vi "TDS RF Signal Output Frequency.vi"(8 "error in (no error)":errorcluster, 9 "Frequency":dbl, 10 "Signal InstConfig":string, 11 "Address":string) -> (0 "error out":errorcluster)   [LabVIEW 2025, in "Interface Functions.lvlib"]
uses:
  Interface Functions.lvlib
panel:
  out "read buffer":string
  # "RF Signal Output Frequency"
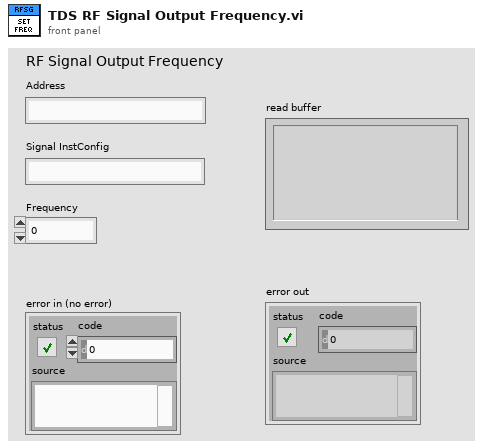
[diagram p1: front panel]
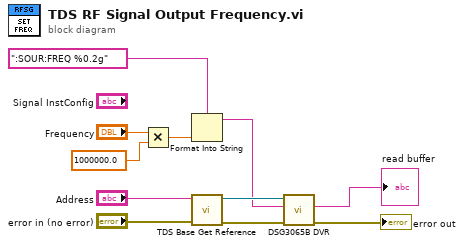
[diagram p0: block diagram]
diagram:
  n1 = Multiply(x="Frequency", y=1000000.0) -> (x*y=w1:dbl)
  n2 = Format Into String(format string=":SOUR:FREQ %0.2g", w1) -> (resulting string=w5:string)  [unwired: 2 in, 1 out]
  n3 = call "TDS Base Get Reference.vi"("error in (no error)"="error in (no error)", "Address"="Address") -> ("error out"=w8:errorcluster, "Reference"=w6:refnum<visa-resource-name>)  [unwired: 8 in]
  n4 = call "DSG3065B DVR.vi"("error in (no error)"=w8, "write buffer"=w5, "VISA resource name"=w6) -> ("error out"=→"error out":errorcluster, "read buffer"=→"read buffer":string)  [unwired: 7 in]
